vi "Write Network Settings.vi"(8 "error in (no error)":errorcluster, 11 "Item Ref":T1=18446744073709551615 format="%.0x") -> (0 "error out":errorcluster)   [LabVIEW 2016, in "Vires VTD System Explorer.lvlib"]
uses:
  Vires VTD System Explorer.lvlib
  <vilib>/NI Veristand/Custom Device API/Custom Device Item Ref.ctl
  <vilib>/NI Veristand/Custom Device API/Custom Device API.lvlib
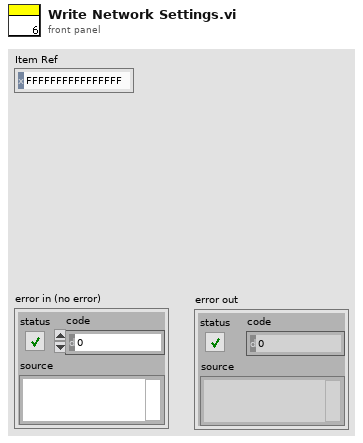
[diagram p1: front panel]
types:
  T1 = typedef "Custom Device API.lvlib/Custom Device Item Ref.ctl" = u64
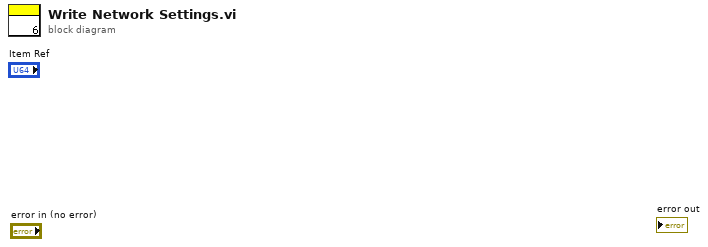
[diagram p0: block diagram]
diagram:
